vi "Initialize Alarm Time Array.vi"(10 "Alarms Time Array in":T1(array[cluster]), 11 "data":waveform(dbl)[](array[waveform])) -> (3 "Alarms Time Array out":T1(array[cluster]))   [LabVIEW 2021, in "DAQ.lvlib"]
uses:
  DAQ.lvlib
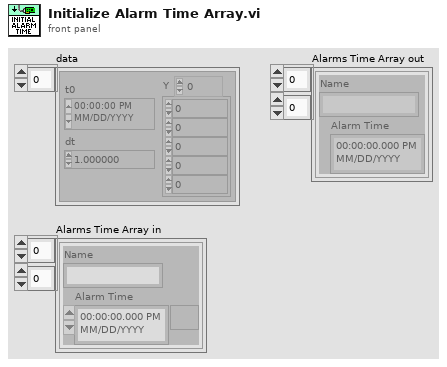
[diagram p1: front panel]
types:
  T1 = cluster{"Name":string, "Alarm Time":timestamp}[][]
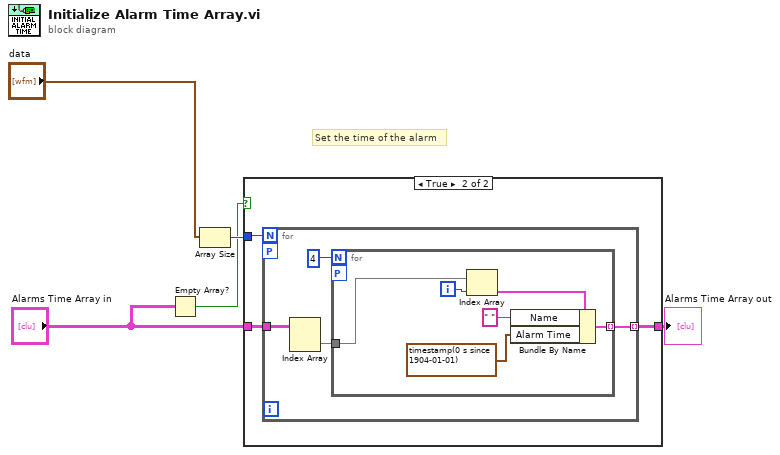
[diagram p0: block diagram]
diagram:
  # "Set the time of the alarm"
  n1 = Empty Array?(array="Alarms Time Array in") -> (empty?=w1:bool)
  n2 = Array Size(array="data") -> (size(s)=w4:i32)
  n3 = case shown="True" w1 {
    tunnel: w4 -> [_ w7]
    tunnel: "Alarms Time Array in" -> [w6 w9]
    tunnel: [w6 w8] -> w5
    frame False {
    }
    frame True {
      n4 = for {
        N: w7 -> [_]
        tunnel: w9 -> [w13]
        tunnel: [w11] -> w8 mode=indexing
        workers-P: _ -> [_]
        n5 = Index Array(array=w13) -> (element=w12:cluster{"Name":string, "Alarm Time":timestamp}[])  [unwired: 2 in]
        n6 = for {
          N: 4 -> [_]
          tunnel: [w17] -> w11 mode=indexing
          tunnel: w12 -> [w16]
          workers-P: _ -> [_]
          i -> [w15]
          n7 = Index Array(array=w16, index=w15) -> (element=w14:cluster{"Name":string, "Alarm Time":timestamp})
          n8 = Bundle By Name(cluster=w14, "Name"=" ", "Alarm Time"=timestamp(0 s since 1904-01-01)) -> (w17:cluster{"Name":string, "Alarm Time":timestamp})
        }
      }
    }
  }
  "Alarms Time Array out" <- w5
